vi "PSF-Fitting.vi"(0 "Centoid X":dbl format="%.2g", 5 "Centroid Y":dbl format="%.2g", 7 "ROI":i32[][](graph), 12 "''/pix":dbl) -> (2 "Credible?":bool, 6 "PSF Graph":cluster{"PSF X":dbl[], "PSF Y":dbl[]}[](graph), 10 "FitProperties":T1, 14 "Seeing":dbl format="%.2g")   [LabVIEW 2011]
uses:
  <vilib>/Analysis/6fits.llb/Curve Fitting Criteria.ctl
  Polymorphics/Distance(single).vi
  <vilib>/Analysis/NI_AALBase.lvlib
  <vilib>/Analysis/NI_AALPro.lvlib
panel:
  in  "CentreUsed":bool=TRUE
  out "Converged?":bool
  out "Barycen X":dbl format="%.2g"
  out "Barycen Y":dbl format="%.2g"
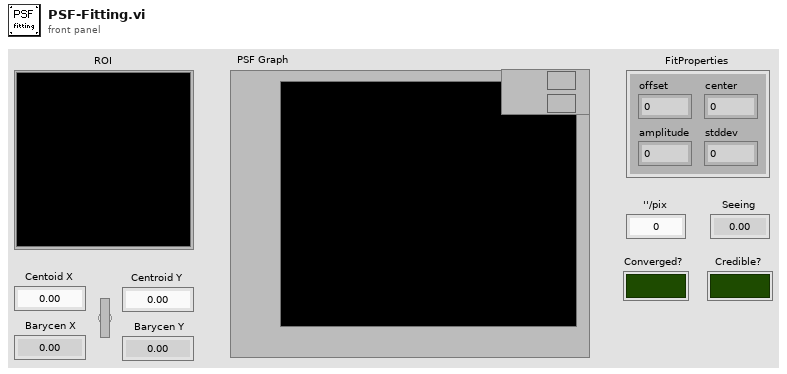
[diagram p1: front panel]
types:
  T1 = cluster{"offset":dbl, "amplitude":dbl, "center":dbl, "stddev":dbl}
  T2 = cluster{"amp min":dbl, "amp max":dbl, "center min":dbl, "center max":dbl, "deviation min":dbl, "deviation max":dbl, "offset min":dbl, "offset max":dbl}
  T3 = typedef "NI_AALPro.lvlib/Curve Fitting Criteria.ctl" = u16
  T4 = cluster{dbl, "center min":dbl, "center min":dbl, "center min":dbl}
  T5 = cluster{"offset":dbl, "amplitude":dbl, "center":dbl, "standard deviation":dbl}
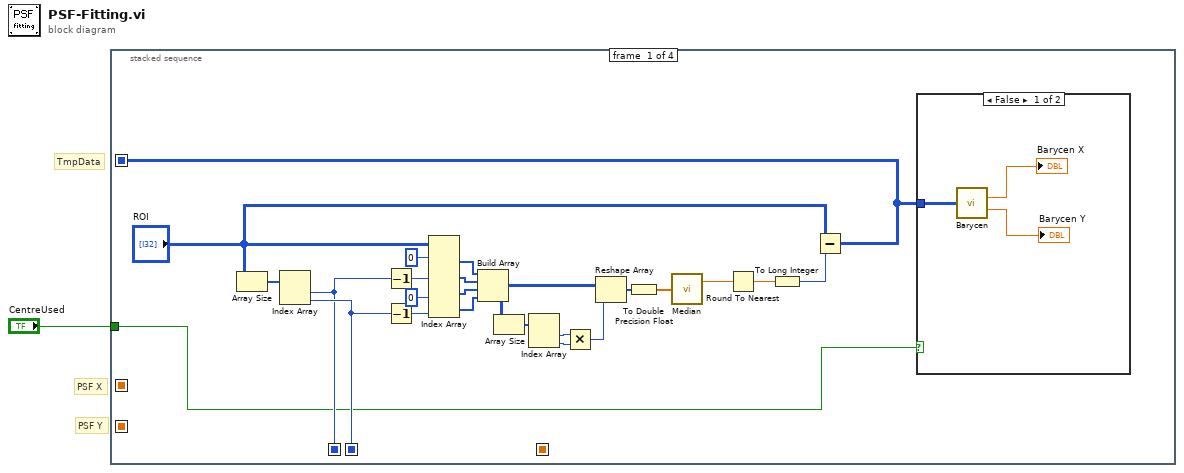
[diagram p0: block diagram]
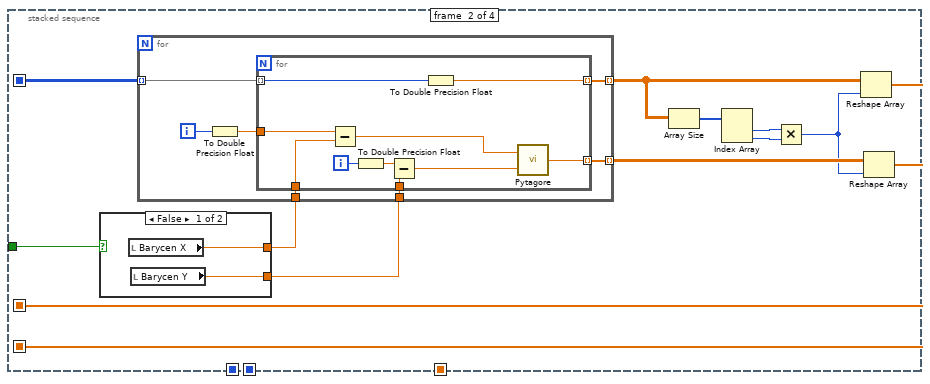
[diagram p3: hidden frame]
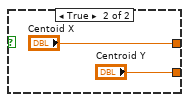
[diagram p4: hidden frame]
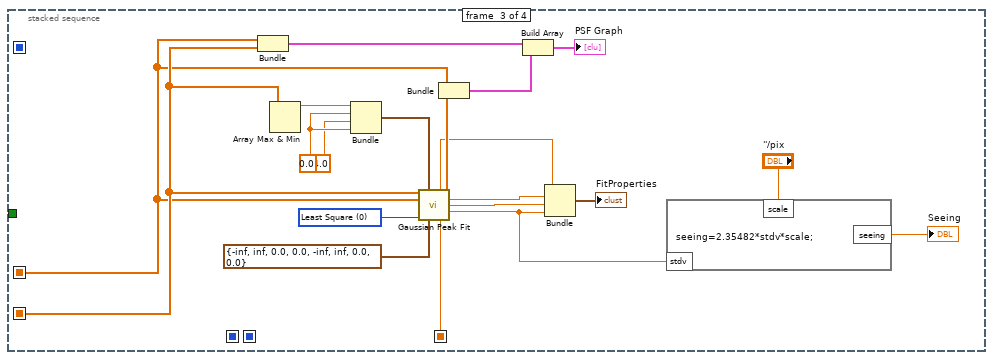
[diagram p5: hidden frame]
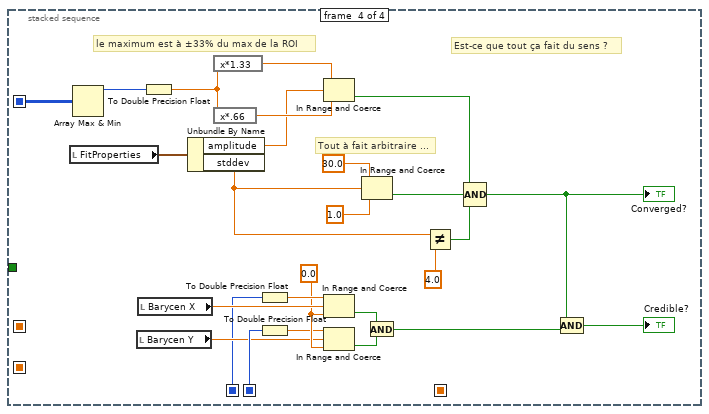
[diagram p6: hidden frame]
diagram:
  # "PSF X"
  # "PSF Y"
  # "TmpData"
  n1 = stacked-sequence {
    seq-local: [w6 _ _ _] -> [_ w34 _ w101]
    seq-local: [_ w32 _ _] -> [_ _ w63 _]
    seq-local: [_ w33 _ _] -> [_ _ w64 _]
    seq-local: [w4 _ _ _] -> [_ _ _ w91]
    seq-local: [w5 _ _ _] -> [_ _ _ w105]
    seq-local: [_ _ w65 _] -> [_ _ _ _]
    tunnel: "CentreUsed" -> [w2 w29 _ _]
    frame #0 {
      n2 = Array Size(array="ROI") -> (size(s)=w10:i32[])
      n3 = Index Array(array=w10) -> (element #1=w4:i32, element #2=w5:i32)  [unwired: 2 in]
      n4 = Decrement(x=w4) -> (x-1=w12:i32)
      n5 = Decrement(x=w5) -> (x-1=w13:i32)
      n6 = Index Array(array="ROI", index (row) #1=0, index (row) #2=w12, index (col) #3=0, index (col) #4=w13) -> (element #1=w18:i32[], element #2=w17:i32[], element #3=w16:i32[], element #4=w15:i32[])  [unwired: 4 in]
      n7 = Build Array(w18, w17, w16, w15) -> (w22:i32[][])
      n8 = Array Size(array=w22) -> (size(s)=w19:i32[])
      n9 = Index Array(array=w19) -> (element #1=w20:i32, element #2=w21:i32)  [unwired: 2 in]
      n10 = Multiply(x=w20, y=w21) -> (x*y=w23:i32)
      n11 = Reshape Array(w22, w23) -> (w24:i32[])
      n12 = To Double Precision Float(number=w24) -> (double precision float=w25:dbl[])
      n13 = call <vilib>:"Median.vi"("X"=w25) -> ("median"=w8:dbl)  [unwired: 1 out]
      n14 = Round To Nearest(number=w8) -> (nearest integer value=w9:dbl)
      n15 = To Long Integer(number=w9) -> (32bit integer=w7:i32)
      n16 = Subtract(x="ROI", y=w7) -> (x-y=w6:i32[][])
      n17 = case shown="False" w2 {
        tunnel: w6 -> [w26 _]
        frame False {
          n18 = call "Barycen.vi"("Array"=w26) -> ("X?"=→"Barycen X":dbl, "Y?"=→"Barycen Y":dbl)  [unwired: 13 in]
        }
        frame True {
        }
      }
    }
    frame #1 {
      n19 = case shown="False" w29 {
        tunnel: [w42 "Centoid X"] -> w31
        tunnel: [w41 "Centroid Y"] -> w30
        frame False {
          n20 = local read "Barycen X"() -> (w42:dbl)
          n21 = local read "Barycen Y"() -> (w41:dbl)
        }
        frame True {
        }
      }
      n22 = for {
        tunnel: w34 -> [w51] mode=indexing
        tunnel: [w50] -> w40 mode=indexing
        tunnel: [w49] -> w39 mode=indexing
        tunnel: w30 -> [w46]
        tunnel: w31 -> [w45]
        i -> [w48]
        n23 = To Double Precision Float(number=w48) -> (double precision float=w47:dbl)
        n24 = for {
          tunnel: w51 -> [w59] mode=indexing
          tunnel: w47 -> [w61]
          tunnel: [w60] -> w50 mode=indexing
          tunnel: [w58] -> w49 mode=indexing
          tunnel: w46 -> [w53]
          tunnel: w45 -> [w52]
          i -> [w57]
          n25 = Subtract(x=w61, y=w52) -> (x-y=w55:dbl)
          n26 = To Double Precision Float(number=w57) -> (double precision float=w56:dbl)
          n27 = Subtract(x=w56, y=w53) -> (x-y=w54:dbl)
          n28 = To Double Precision Float(number=w59) -> (double precision float=w58:dbl)
          n29 = call-poly "Pytagore.vi"("D2"=w54, "D1"=w55) -> ("DT"=w60:dbl)
        }
      }
      n30 = Array Size(array=w39) -> (size(s)=w38:i32[])
      n31 = Index Array(array=w38) -> (element #1=w37:i32, element #2=w36:i32)  [unwired: 2 in]
      n32 = Multiply(x=w37, y=w36) -> (x*y=w35:i32)
      n33 = Reshape Array(w39, w35) -> (w33:dbl[])
      n34 = Reshape Array(w40, w35) -> (w32:dbl[])
    }
    frame #2 {
      w73 = T3 0 items=["Least Square", "Least Absolute Residual", "Bisquare"] ("method")
      w76 = 0.0 ("center min")
      n35 = Bundle(w63, w64) -> (w80:cluster{dbl[], dbl[]})  [unwired: 1 in]
      n36 = Array Max & Min(array=w64) -> (max value=w77:dbl)  [unwired: 3 out]
      n37 = Bundle(w77, "center min"=w76, "center min"=4.0, "center min"=w76) -> (w74:T4)  [unwired: 1 in]
      n38 = call <vilib>:"Gaussian Peak Fit.vi"("Y"=w64, "initial guess"=w74, "X"=w63, "method"=w73, "parameter bounds"=T2 {"amp min"=-inf, "amp max"=inf, "center min"=0.0, "center max"=0.0, "deviation min"=-inf, "deviation max"=inf, "offset min"=0.0, "offset max"=0.0}) -> ("offset"=w69:dbl, "Best Gaussian Fit"=w78:dbl[], "amplitude"=w72:dbl, "center"=w71:dbl, "standard deviation"=w66:dbl, "residue"=w65:dbl)  [unwired: 4 in, 1 out]
      n39 = Bundle(w63, "Best Gaussian Fit"=w78) -> (w81:cluster{dbl[], "Best Gaussian Fit":dbl[]})  [unwired: 1 in]
      n40 = Build Array(w80, w81) -> (→"PSF Graph":cluster{dbl[], "Best Gaussian Fit":dbl[]}[])
      n41 = Bundle("offset"=w69, "amplitude"=w72, "center"=w71, "standard deviation"=w66) -> (→"FitProperties":T5)  [unwired: 1 in]
      n42 = formula code="seeing=2.35482*stdv*scale;"("stdv"=w66, "scale"="''/pix") -> ("seeing"=→"Seeing":dbl)
    }
    frame #3 {
      w104 = 0.0 ("lower limit")
      # "Tout à fait arbitraire ..."
      # "le maximum est à ±33% du max de la ROI"
      # "Est-ce que tout ça fait du sens ?"
      n43 = local read "FitProperties"() -> (w100:T1)
      n44 = Array Max & Min(array=w101) -> (max value=w99:i32)  [unwired: 3 out]
      n45 = local read "Barycen Y"() -> (w92:dbl)
      n46 = local read "Barycen X"() -> (w107:dbl)
      n47 = To Double Precision Float(number=w99) -> (double precision float=w98:dbl)
      n48 = Unbundle By Name(w100) -> ("amplitude"=w95:dbl, "stddev"=w84:dbl)
      n49 = expression code="x*1.33"(w98) -> (w96:dbl)
      n50 = expression code="x*.66"(w98) -> (w97:dbl)
      n51 = To Double Precision Float(number=w91) -> (double precision float=w106:dbl)
      n52 = To Double Precision Float(number=w105) -> (double precision float=w93:dbl)
      n53 = In Range and Coerce(upper limit=w96, x=w95, lower limit=w97) -> (In Range?=w87:bool)  [unwired: 1 out]
      n54 = In Range and Coerce(upper limit=w106, x=w107, lower limit=w104) -> (In Range?=w103:bool)  [unwired: 1 out]
      n55 = In Range and Coerce(upper limit=w93, x=w92, lower limit=w104) -> (In Range?=w102:bool)  [unwired: 1 out]
      n56 = In Range and Coerce(upper limit=30.0, x=w84, lower limit=1.0 ("upper limit")) -> (In Range?=w85:bool)  [unwired: 1 out]
      n57 = And(x=w103, y=w102) -> (x .and. y?=w88:bool)
      n58 = Not Equal?(x=w84, y=4.0) -> (x != y?=w83:bool)
      n59 = Compound Arithmetic op=AND(w87, w85, w83) -> (w86:bool)
      "Converged?" <- w86
      n60 = Compound Arithmetic op=AND(w86, w88) -> (→"Credible?":bool)
    }
  }
